vi "Stop Core.vi"(10 "final error code":i32, 11 "GameLogic in":refnum<class "GameLogic.lvclass">) -> (3 "GameLogic out":refnum<class "GameLogic.lvclass">)   [LabVIEW 2019, in "GameLogic.lvlib" / "GameLogic.lvclass"]
doc: "(<B>Filename</B>: Actor Framework.lvlib:Actor.lvclass:Stop Core.vi)\n\nDefines what the actor does before it stops. Use the <B>final error code</B> input to determine whether the actor shut down in response to an error.\n\nBy default, this method passes the Stop message along to all auto-stop nested actors. A descendant class may override this method to define additional behavior, such as shutting down any processes the actor initiated in its override of the Actor Core method."
uses:
  GameLogic.lvclass
  GameLogic.lvclass/GameLogic.ctl
  <vilib>/ActorFramework/Actor/Actor.lvclass
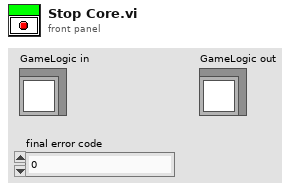
[diagram p1: front panel]
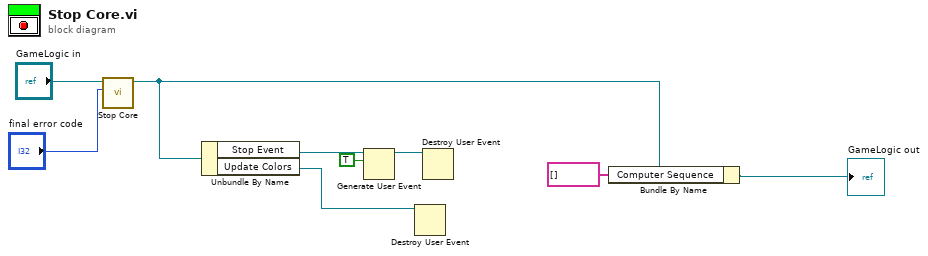
[diagram p0: block diagram]
diagram:
  n1 = call-parent "Stop Core.vi"("final error code"="final error code", "Actor in"="GameLogic in") -> ("Actor out"=w3:refnum<class "GameLogic.lvclass">)  [unwired: 9 in]
  n2 = Unbundle By Name(w3) -> ("Stop Event"=w7:refnum<user-event>, "Update Colors"=w6:refnum<user-event>)
  n3 = Generate User Event(user event=w7, event data cluster=TRUE ("event data")) -> (user event out=w5:refnum<user-event>)  [unwired: 2 in, 1 out]
  n4 = Destroy User Event(user event=w6) -> ()  [unwired: 1 in, 1 out]
  n5 = Destroy User Event(user event=w5) -> ()  [unwired: 1 in, 1 out]
  n6 = Bundle By Name(cluster=w3, "Computer Sequence"=string[] []) -> (→"GameLogic out":refnum<class "GameLogic.lvclass">)
